vi "Uniquify_Label.vi"(8 "error in (no error)":errorcluster, 10 "names":string[](array[string]), 11 "userFolder in":refnum<class "userFolder.lvclass">) -> (0 "error out":errorcluster, 2 "name":string, 3 "userFolder out":refnum<class "userFolder.lvclass">)   [LabVIEW 2020, in "userFolder.lvclass"]
uses:
  <vilib>/AppBuilder/IB_Classes/Destination/userFolder/userFolder.lvclass
  <vilib>/AppBuilder/IB_Classes/Destination/userFolder/userFolder.lvclass/userFolder.ctl
  <resource>/Framework/Providers/Builds/Installer/CDK_GLOBAL_STRINGS.vi
  <vilib>/AppBuilder/IB_Classes/Destination/IB_Destination.lvclass
  e:/builds/penguin/labview/branches/2020/dev/dist/vi.lib/AppBuilder/IB_Classes/Destination/IB_Destination.lvclass
  e:/builds/penguin/labview/branches/2020/dev/dist/vi.lib/AppBuilder/IB_Classes/Destination/userFolder/userFolder.lvclass
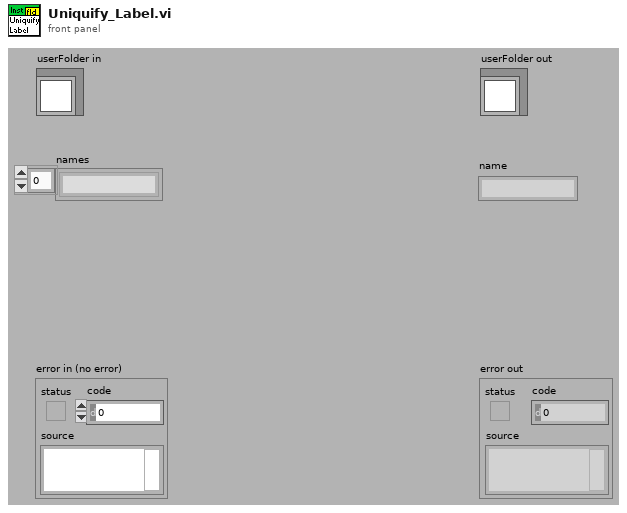
[diagram p1: front panel]
types:
  T1 = typedef "IB_Destination.ctl" = cluster{"name":string, "unlock":bool, "parentTag":string, "destTag":string, "eng_installPath":string}
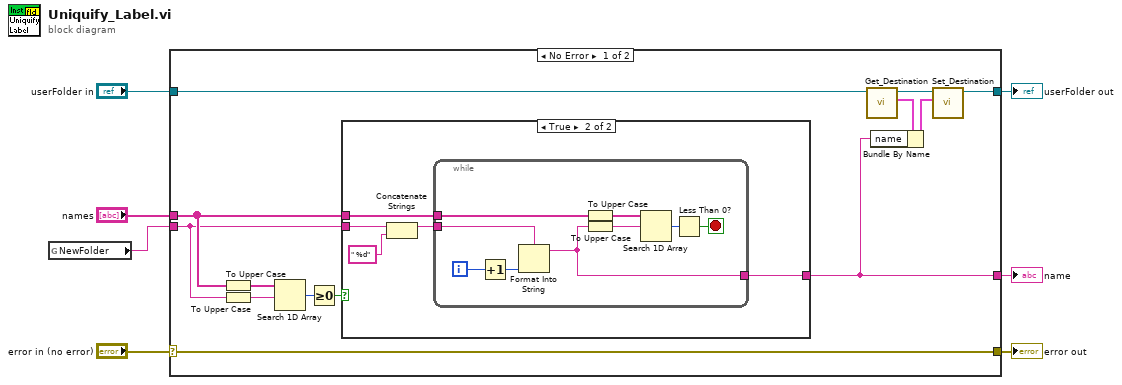
[diagram p0: block diagram]
diagram:
  n1 = global read "CDK_GLOBAL_STRINGS.vi" "NewFolder"() -> (w6:string)
  n2 = case shown="No Error" "error in (no error)" {
    selector: "error in (no error)" -> [w20 w37]
    tunnel: [w20 w37] -> w4
    tunnel: "names" -> [w15 _]
    tunnel: w6 -> [w14 _]
    tunnel: [w10 _] -> w3
    tunnel: "userFolder in" -> [w9 w36]
    tunnel: [w8 w36] -> w1
    frame No Error {
      n3 = To Upper Case(1:w15) -> (0:w17:string[])
      n4 = To Upper Case(1:w14) -> (0:w16:string)
      n5 = Search 1D Array(1D array=w17, element=w16) -> (index of element=w19:i32)  [unwired: 1 out]
      n6 = Greater Or Equal To 0?(x=w19) -> (x >= 0?=w18:bool)
      n7 = case shown="True" w18 {
        tunnel: w15 -> [_ w26]
        tunnel: w14 -> [w21 w25]
        tunnel: [w21 w22] -> w10
        frame False {
        }
        frame True {
          n8 = Concatenate Strings(w25, " %d" ("string")) -> (w23:string)
          n9 = while {
            tunnel: w26 -> [w31]
            tunnel: w23 -> [w33]
            tunnel: [w29] -> w22
            i -> [w27]
            stop <- w34 stop-if-true
            n10 = Increment(x=w27) -> (x+1=w28:i32)
            n11 = Format Into String(format string=w33, w28) -> (resulting string=w29:string)  [unwired: 2 in, 1 out]
            n12 = To Upper Case(1:w31) -> (0:w32:string[])
            n13 = To Upper Case(1:w29) -> (0:w30:string)
            n14 = Search 1D Array(1D array=w32, element=w30) -> (index of element=w35:i32)  [unwired: 1 out]
            n15 = Less Than 0?(x=w35) -> (x < 0?=w34:bool)
          }
        }
      }
      n16 = call <vilib>:"Get_Destination.vi"("IB_Destination in"=w9) -> ("data"=w12:T1, "IB_Destination out"=w13:refnum<class "userFolder.lvclass">)  [unwired: 1 in, 8 out]
      n17 = Bundle By Name(cluster=w12, "name"=w10) -> (w11:T1)
      n18 = call <vilib>:"Set_Destination.vi"("data"=w11, "IB_Destination in"=w13) -> ("IB_Destination out"=w8:refnum<class "userFolder.lvclass">)  [unwired: 1 in, 8 out]
    }
    frame Error {
    }
  }
  "error out" <- w4
  "userFolder out" <- w1
  "name" <- w3
